vi "Pivot Immediate_wrapper.vi"() -> ()   [LabVIEW 2025]
uses:
  <vilib>/Rock Robotics/WPI/Framework/Command Status Info.ctl
  <vilib>/Rock Robotics/WPI/Framework/Completion Status.ctl
  <vilib>/Rock Robotics/WPI/Framework/Completion Notifier.ctl
  Implementation/Pivot Operations.ctl
panel:
  out "Command Info Out":T1
  in  "Setpoint":dbl
  in  "Operation":T4
  in  "Command Info In":T1
  in  "Description":string
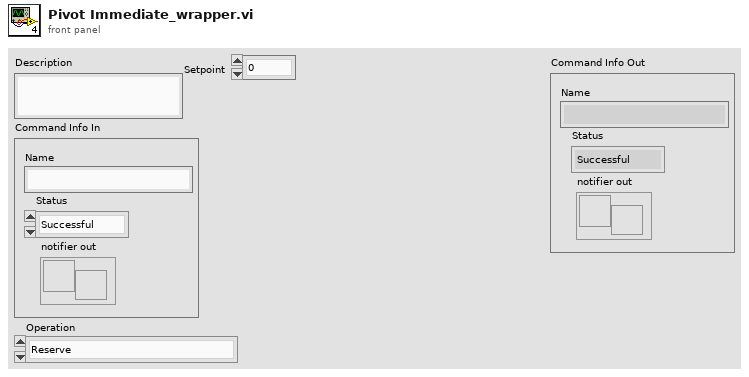
[diagram p1: front panel]
types:
  T1 = typedef "Command Status Info.ctl" = cluster{"Name":string, "Status":T2, "notifier out":T3}
  T2 = typedef "Completion Status.ctl" = enum16{"Successful", "Aborted", "Incomplete"}
  T3 = typedef "Completion Notifier.ctl" = refnum<notifier>
  T4 = typedef "Pivot Operations.ctl" = enum16{"Reserve", "Read Current", "Retract Pivot", "Extend Pivot", "Reset Pivot", "Immediate", "Extend Pivot Auto"}
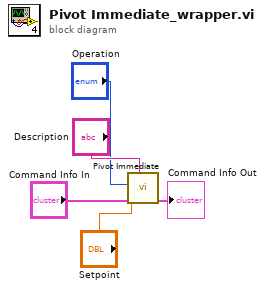
[diagram p0: block diagram]
diagram:
  n1 = call "Pivot Immediate.vi"("Description"="Description", "Command Info In"="Command Info In", "Operation"="Operation", "Setpoint"="Setpoint") -> ("Command Info Out"=→"Command Info Out":T1)  [unwired: 7 in]
